vi "GOOP_GetMenuPlugins.vi"() -> (1 "MenuPluginsVIs":path[](array[path]), 2 "MenuPlugins(E.g. GOOP/My function)":string[](array[string]))   [LabVIEW 2014]
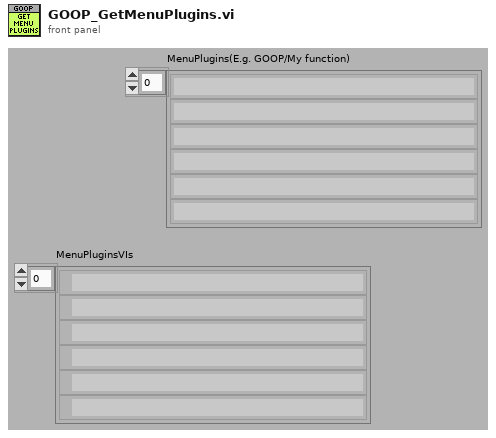
[diagram p1: front panel]
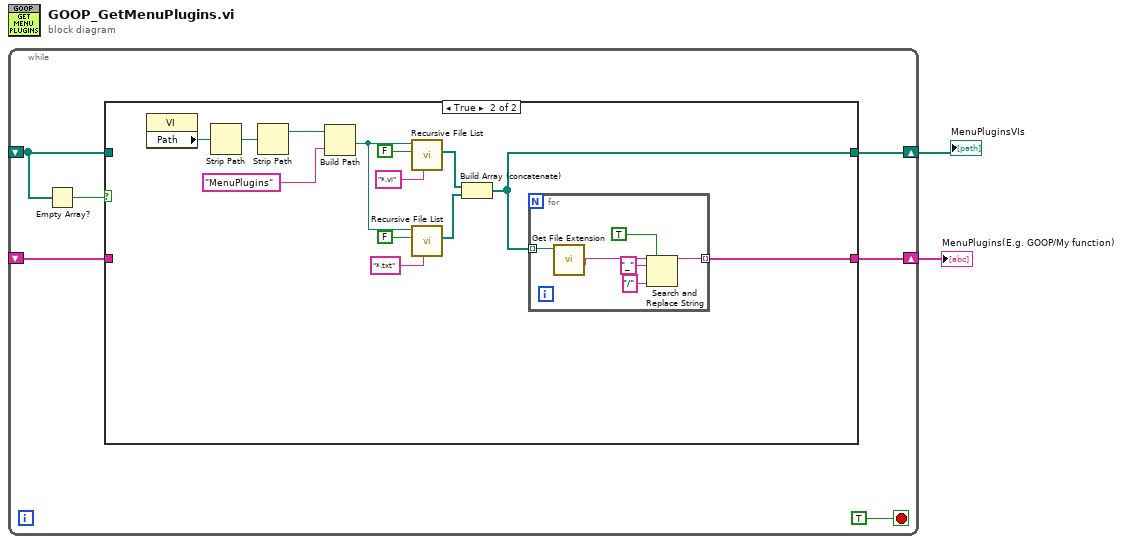
[diagram p0: block diagram]
diagram:
  n1 = while {
    shift-right: [w5] -> w2
    shift-left: _ -> [w6]
    shift-right: [w3] -> w1
    shift-left: _ -> [w4]
    stop <- TRUE stop-if-true
    n2 = Empty Array?(array=w6) -> (empty?=w7:bool)
    n3 = case shown="True" w7 {
      tunnel: w6 -> [w10 _]
      tunnel: [w10 w11] -> w5
      tunnel: w4 -> [w9 _]
      tunnel: [w9 w18] -> w3
      frame False {
      }
      frame True {
        n4 = property class="VI"() -> ("Path"=w23:path)  [unwired: 2 in, 2 out]
        n5 = Strip Path(path=w23) -> (stripped path=w22:path)  [unwired: 1 out]
        n6 = Strip Path(path=w22) -> (stripped path=w21:path)  [unwired: 1 out]
        n7 = Build Path(base path=w21, name or relative path="MenuPlugins") -> (appended path=w14:path)
        n8 = call <vilib>:"Recursive File List.vi"("pattern"="*.vi", "Treat LLBs as Folders?"=FALSE, "Folder Path"=w14) -> ("All Files in Dir"=w12:path[])  [unwired: 4 in, 4 out]
        n9 = call <vilib>:"Recursive File List.vi"("pattern"="*.txt", "Treat LLBs as Folders?"=FALSE, "Folder Path"=w14) -> ("All Files in Dir"=w13:path[])  [unwired: 4 in, 4 out]
        n10 = Build Array (concatenate)(w12, w13) -> (w11:path[])
        n11 = for {
          tunnel: w11 -> [w25] mode=indexing
          tunnel: [w26] -> w18 mode=indexing
          n12 = call <vilib>:"Get File Extension.vi"("file"=w25) -> ("filename without extension"=w24:string)  [unwired: 7 in, 3 out]
          n13 = Search and Replace String(replace all?=TRUE ("replace all? (F)"), input string=w24, search string="_", replace string="/" ("replace string (\"\")")) -> (result string=w26:string)  [unwired: 4 in, 3 out]
        }
      }
    }
  }
  "MenuPlugins(E.g. GOOP/My function)" <- w1
  "MenuPluginsVIs" <- w2
